vi "Check Escala.vi"(8 "error in (no error)":errorcluster, 10 "Grandeza":string, 11 "U1213A in":refnum<class "U1213A.lvclass">) -> (0 "error out":errorcluster, 2 "Escala Correta?":bool, 3 "U1213A out":refnum<class "U1213A.lvclass">)   [LabVIEW 2015, in "U1213A.lvclass"]
uses:
  U1213A.lvclass
  <instrlib>/U1250 Series Multimeter Device Driver/U1250 Series Digital Multimeter.lvlib
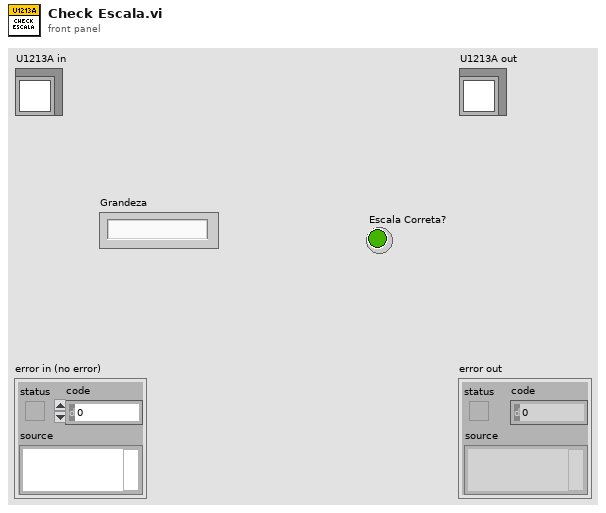
[diagram p1: front panel]
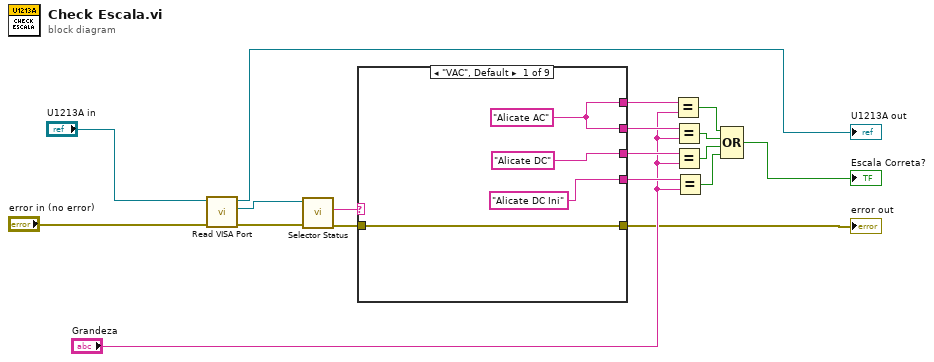
[diagram p0: block diagram]
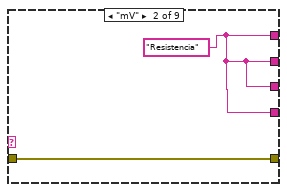
[diagram p2: hidden frame]
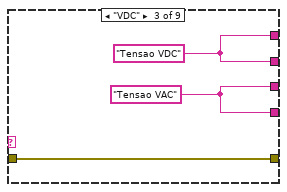
[diagram p3: hidden frame]
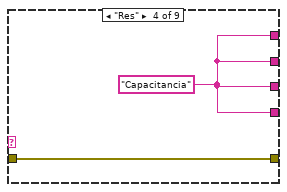
[diagram p4: hidden frame]
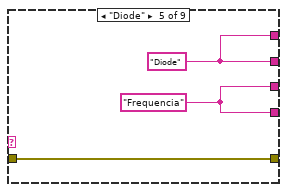
[diagram p5: hidden frame]
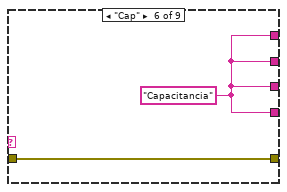
[diagram p6: hidden frame]
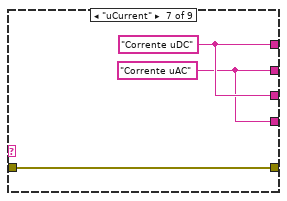
[diagram p7: hidden frame]
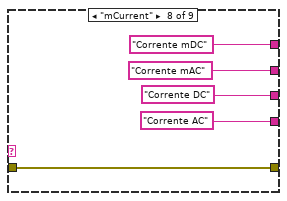
[diagram p8: hidden frame]
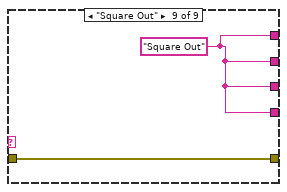
[diagram p9: hidden frame]
diagram:
  n1 = call-dynamic "Read VISA Port.vi"("error in (no error)"="error in (no error)", "Device in"="U1213A in") -> ("error out"=w18:errorcluster, "VISA Port"=w1:refnum<visa-resource-name>, "Device out"=→"U1213A out":refnum<class "U1213A.lvclass">)  [unwired: 7 in]
  n2 = call <instrlib>:"Selector Status.vi"("error in (no error)"=w18, "VISA resource name"=w1) -> ("error out"=w15:errorcluster, "Selector Option"=w17:string)  [unwired: 7 in, 1 out]
  n3 = case shown="\"VAC\", Default" w17 {
    tunnel: [w21 w23 w26 w28 w31 w33 w35 "Corrente mAC" w43] -> w16
    tunnel: [w22 w24 w27 w29 w32 w34 w37 w41 w44] -> w4
    tunnel: w15 -> [w22 w24 w27 w29 w32 w34 w37 w41 w44]
    tunnel: [w21 w23 w26 w28 w31 w33 w36 "Corrente mDC" w43] -> w13
    tunnel: ["Alicate DC" w23 w25 w28 w30 w33 w36 "Corrente DC" w43] -> w11
    tunnel: ["Alicate DC Ini" w23 w25 w28 w30 w33 w35 "Corrente AC" w43] -> w10
    frame "VAC", Default {
      w21 = "Alicate AC"
    }
    frame "mV" {
      w23 = "Resistencia"
    }
    frame "VDC" {
      w25 = "Tensao VAC"
      w26 = "Tensao VDC"
    }
    frame "Res" {
      w28 = "Capacitancia"
    }
    frame "Diode" {
      w30 = "Frequencia"
      w31 = "Diode"
    }
    frame "Cap" {
      w33 = "Capacitancia"
    }
    frame "uCurrent" {
      w36 = "Corrente uDC"
      w35 = "Corrente uAC"
    }
    frame "mCurrent" {
    }
    frame "Square Out" {
      w43 = "Square Out"
    }
  }
  "error out" <- w4
  n4 = Equal?(x=w13, y="Grandeza") -> (x = y?=w14:bool)
  n5 = Equal?(x=w16, y="Grandeza") -> (x = y?=w12:bool)
  n6 = Equal?(x=w11, y="Grandeza") -> (x = y?=w8:bool)
  n7 = Equal?(x=w10, y="Grandeza") -> (x = y?=w9:bool)
  n8 = Compound Arithmetic op=OR(w14, w12, w8, w9) -> (→"Escala Correta?":bool)
